vi "Demo.vi"() -> ()   [LabVIEW 2011]
panel:
  in  "Rows and Cols":i32[](array[numeric])=[3, 3]
  in  "Start Point":cluster{"x":i16, "y":i16}={"x"=50, "y"=50} caption="Start (x,y)"
  in  "Para":T1={"Frame?"=TRUE, "Pen and Color"={"pen"={"Width"=4, "Style"=enum."Solid"}, "color(black)"=0}}
  in  "Image File Path":path=path "E:/BOOK/功能块/图片工具/Pic to RGB Channel/demoPic3.jpg"
  out "Picture out":picture
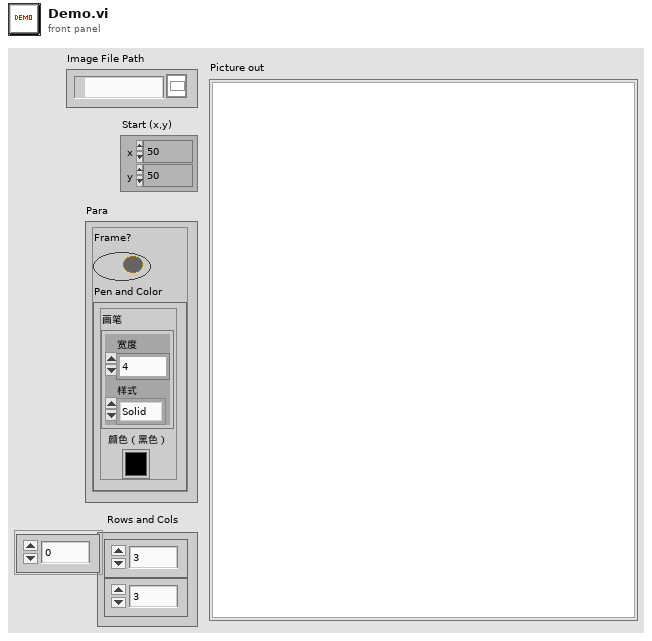
[diagram p1: front panel]
types:
  T1 = cluster{"Frame?":bool, "Pen and Color":cluster{"pen":cluster{"Width":i16, "Style":enum32{"Solid", "Dash", "Dot", "DashDot", "DashDotDot"}}, "color(black)":u32}}
  T2 = typedef "imagedata.ctl" = cluster{"image type":i32, "image depth":i32, "image":u8[], "mask":u8[], "colors":u32[], "Rectangle":cluster{"left":i16, "top":i16, "right":i16, "bottom":i16}}
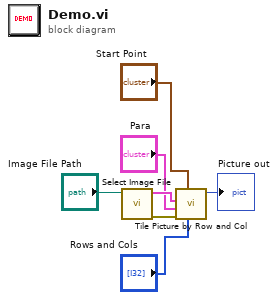
[diagram p0: block diagram]
diagram:
  n1 = call "Select Image File.vi"("文件路径输入控件"="Image File Path") -> ("error out"=w6:errorcluster, "image data"=w5:T2)  [unwired: 9 in]
  n2 = call "Tile Picture by Row and Col.vi"("Rows and Cols"="Rows and Cols", "Start Point"="Start Point", "错误输入"=w6, "Para"="Para", "image data"=w5) -> ("Picture out"=→"Picture out":picture)  [unwired: 5 in, 1 out]
